vi "Dashboard Main.vi"() -> ()   [LabVIEW 2015]
uses:
  <vilib>/Utility/miscctls.llb/LVRowAndColumnTypeDef.ctl
  <vilib>/event_ctls.llb/eventvkey.ctl
  <vilib>/Rock Robotics/WPI/Dashboard/WPI_DashboardLogging Global.vi
  <vilib>/Rock Robotics/Network Tables/NT Read Numeric Array.vi
  <vilib>/Rock Robotics/Network Tables/NT Write Boolean.vi
  <vilib>/Utility/config.llb/Write Key (String).vi
  <vilib>/Utility/config.llb/Write Key (I32).vi
  <vilib>/Utility/config.llb/NI_LVConfig.lvlib
panel:
  in  "TCP":refnum<k5>
  in  "Rec Mode":enum32{"Stop", "Record", "Playback"}(radio)
  in  "Vision":u16(ring) items=["Camera Off", "USB Camera SW", "USB Camera HW", "IP Camera"]
  out "Camera IP":string
  out "Image Message":string="Timeout in Camera Communications"
  in  "Dashboard Tab":T1(tab)
  out "RPMs":dbl
  in  "Select Auto":string(combo)
  out "NT Connection":bool
  in  "Camera Settings":T2={"Frame Rate"=30, "Compression"=30, "Size"=1} {"Frame Rate" scale=1.0..30.0; "Size" items=["640x480", "320x240", "160x120"]}
  out "MotorChart R":cluster{"Numeric":dbl, "Numeric":dbl}(graph)
  out "MotorChart L":T3(graph)
  out "MotorSliders R":cluster{"MotorSlide1":dbl, "MotorSlide2":dbl} {"MotorSlide2" scale=-1.0..1.0 scale format="%#_2e"; "MotorSlide1" scale=-1.0..1.0 scale format="%#_2e"}
  out "MotorSliders L":T4 {"MotorSlide4 2" scale=0.0..14.0 scale format="%#_2e"; "MotorSlide2" scale=-1.0..1.0 scale format="%#_2e"; "MotorSlide1" scale=-1.0..1.0 scale format="%#_2e"}
  out "Gyro":dbl(knob) scale=0.0..360.0
  out "JS1 Z":dbl(slide) scale=-1.0..1.0 scale format="%#_2e"
  out "JS1 Graph":cluster{"X":dbl, "Y":dbl}[](graph)
  out "JS1 Buttons":T5
  out "JS2 Z":dbl(slide) scale=-1.0..1.0 scale format="%#_2e"
  out "JS2 Graph":cluster{"X":dbl, "Y":dbl}[](graph)
  out "JS2 Buttons":T5
  out "Mode":T6(ring)=enum."Auto Disabled"
  in  "DB Camera Config":bool
  out "fps":dbl format="%#.1g"
  out "Mbps":dbl format="%#.1g"
  out "Mbps LED":bool
  out "Particles (F)":dbl
  in  "Dispose Vision":bool
  out "Particles (M)":dbl
  in  "Load File":bool
  in  "Color Components":T7={"Hue"={8.0, 168.0}, "Sat"={21.0, 255.0}, "Val"={229.0, 255.0}} {"Val" scale=0.0..255.0; "Sat" scale=0.0..255.0; "Hue" scale=0.0..255.0 scale format="%#_3g"}
  in  "DB/String 9":string
  in  "DB/String 8":string
  in  "DB/String 7":string
  in  "DB/String 6":string
  in  "DB/String 5":string
  in  "DB/String 4":string
  in  "DB/String 3":string
  in  "DB/String 2":string
  in  "DB/String 1":string
  in  "DB/String 0":string
  in  "DB/Slider 0":dbl(slide) scale=0.0..5.0
  in  "DB/Slider 1":dbl(slide) scale=0.0..5.0
  in  "DB/Slider 2":dbl(slide) scale=0.0..5.0
  in  "DB/Slider 3":dbl(slide) scale=0.0..5.0
  out "DB/LED 3":bool
  out "DB/LED 2":bool
  out "DB/LED 1":bool
  out "DB/LED 0":bool
  in  "DB/Button 3":bool
  in  "DB/Button 2":bool
  in  "DB/Button 1":bool
  in  "DB/Button 0":bool caption="New Name"
  in  "Test Slider":dbl(slide) scale=0.0..100.0 scale format="%#_3g"
  in  "On/Off":bool caption="Solenoid"
  in  "Test Name":u16(ring) items=["Select the test to run..."]
  in  "Test Tree":string(tree)
  in  "Motor":cluster{"Value":dbl, "Enable":bool} {"Value" scale=-1.0..1.0 scale format="%#_3g"}
  out "Progress":T8 {"Test Progress" scale=0.0..100.0}
  in  "Rev/Fwd":cluster{"Forward":bool, "Reverse":bool}
  in  "Test Ring":u16(ring) items=["Monochrome", "Color"]
  out "Cmd Status":string
  in  "Execute Command":bool
  in  "Command Params":string[][](table)
  in  "Command Selection":i32(listbox)
  in  "CheckList":i32(listbox)
  out "Tree":string(tree)
  out "Camera Image":T9(plugin-control)
  out "Background":bool
  # "Left"
  # "Front"
  # "Right"
  # "Battery"
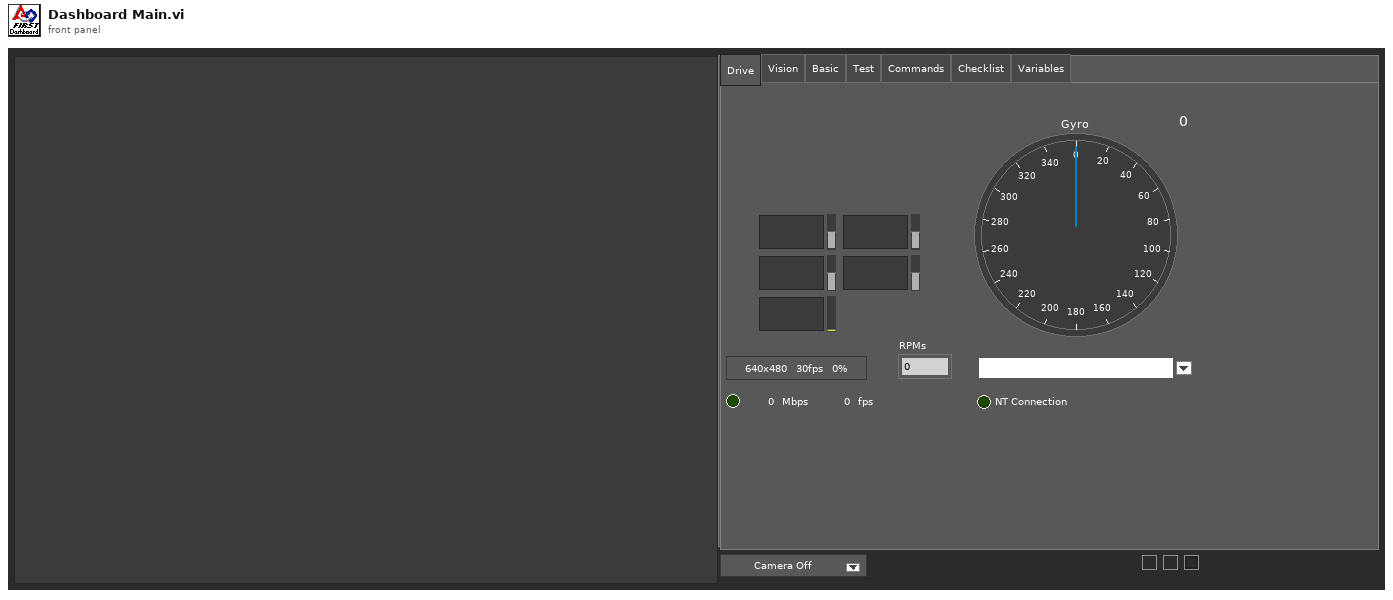
[diagram p1: front panel]
types:
  T1 = enum32{"Drive", "Vision", "Basic", "Test", "Commands", "Checklist", "Variables"}
  T2 = cluster{"Frame Rate":i32, "Compression":i32, "Size":u16}
  T3 = cluster{"Numeric":dbl, "Numeric":dbl, "Battery V":dbl}
  T4 = cluster{"MotorSlide1":dbl, "MotorSlide2":dbl, "MotorSlide4 2":dbl}
  T5 = cluster{bool, bool, bool, bool, bool, bool, bool, bool, bool, bool, bool, bool}
  T6 = enum8{"Tele-Op Disabled", "Tele-Op Enabled", "Auto Disabled", "Auto Enabled", "Test Disabled", "Test Enabled", "Disconnected", "No Code", "E-Stop"}
  T7 = cluster{"Hue":cluster{dbl, dbl}, "Sat":cluster{dbl, dbl}, "Val":cluster{dbl, dbl}}
  T8 = cluster{"Test Progress":u8, "Test Progress Text":string}
  T9 = typedef "IMAQ Image.ctl" = refnum<image>
  T10 = cluster{"IDs":cluster{"RPC field ID":u16, "Unique ID":u16}, "String":string}
  T11 = enum32{"Drive", "Basic", "Custom", "Test", "Checklist", "Variables"}
  T12 = typedef "Image Type" = u32
  T13 = cluster{"Camera Image":refnum<vi>, "Dashboard Tab":refnum<vi>, "Background":refnum<vi>, "Vision":refnum<vi>, "Rec Mode":refnum<vi>, "Test Slider":refnum<vi>, "On/Off ":refnum<vi>, "Test Ring":refnum<vi>, "Rev/Fwd":refnum<vi>, "Test Name":refnum<vi>, "Motor":refnum<vi>, "Progress":refnum<vi>, "CheckList":refnum<vi>, "Tree":refnum<vi>, "Test Tree":refnum<vi>, "Command Params":refnum<vi>, "Command Selection":refnum<vi>, "Execute Command":refnum<vi>, "Cmd Status":refnum<vi>}
  T14 = cluster{"Error Strings":string, "Disable Counts":cluster{u16, u16}, "Rail Faults":cluster{u16, u16, u16}, "Robot IP":string, "DB Mode":u8, "Event Info":cluster{"Name":string, "Type":u8, "Number":u16, "Replay":u8}, "Camera Addr":string}
  T15 = cluster{"Storage":cluster{"Disk Free":u64, "RAM Block":u32, "RAM free":u32}, "CPU Utilization":cluster{"CPU % ISR":sgl, "CPU % Time Crit":sgl, "CPU % Timed Str":sgl, "CPU % High":sgl, "CPU % Above":sgl, "CPU % Normal":sgl, "CPU % Low":sgl}, "CAN":cluster{"% Bus Utilization":sgl, "Bus Off Cnt":u32, "TX_FIFO Full Cnt":u32, "Receive Error Cnt":u8, "Transmit Error Cnt":u8}, "HID":cluster{"HID Outputs":u32, "Rumble Low":u16, "Rumble High":u16}[]}
  T16 = cluster{"Status bits":cluster{"Test Mode":bool, "Autonomous":bool, "Enabled":bool, "Code Start":bool, "Brownout":bool, "Reserved 2":bool, "Reserved 3":bool, "E-Stop":bool}, "Code Trace":cluster{"Disabled":bool, "TeleOp":bool, "Auto":bool, "Test":bool}, "Controller Type":enum16{"unknown", "cRIO", "roboRio"}, "Code?":enum16{"unknown", "noCode", "code"}, "Battery V":dbl}
  T17 = cluster{"Control Bits":cluster{"TestMode":bool, "Autonomous":bool, "Enabled":bool, "FMS Present":bool, bool, bool, bool, "E-Stop":bool}, "Team Station ":u8, "Countdown":sgl, "Joystick Values":cluster{"Axes":dbl[], "Buttons":bool[], "POVs":i16[]}[]}
  T18 = cluster{"Axes":dbl[], "Buttons":bool[], "POVs":i16[]}[]
  T19 = cluster{"Axes":dbl[], "Buttons":bool[], "POVs":i16[]}
  T20 = cluster{"Buttons[0]":bool, "Buttons[1]":bool, "Buttons[2]":bool, "Buttons[3]":bool, "Buttons[4]":bool, "Buttons[5]":bool, "Buttons[6]":bool, "Buttons[7]":bool, "Buttons[8]":bool, "Buttons[9]":bool, "Buttons[10]":bool, "Buttons[11]":bool}
  T21 = cluster{"Left":i32, "Top":i32, "Right":i32, "Bottom":i32}
  T22 = cluster{cluster{dbl, dbl}, cluster{dbl, dbl}, cluster{dbl, dbl}}
  T23 = typedef "NI_LVConfig.lvlib/Config Data RefNum.ctl" = refnum<k1>
  T24 = cluster{"Operation":enum16{"Update", "Clear"}, "Color Box":u32}[]
  T25 = typedef "eventvkey.ctl" = enum16{"ASCII", "Enter", "Return", "Shift", "Ctrl", "Alt", "Cmd", "Opt", "Caps", "NumLock", "Clear", "Break", "Up", "Down", "Left", "Right", "Insert", "Delete", "Home", "End", "PageUp", "PageDown", "Escape", "Help", "Pause", "ScrollLock", "F1", "F2", "F3", "F4", "F5", "F6", "F7", "F8", "F9", "F10", "F11", "F12", "F13", "F14", "F15", "F16", "F17", "F18", "F19", "F20", "F21", "F22", "F23", "F24", "Play", "VolumeUp", "VolumeDown", "Mute", "Two Byte Char"}
  T26 = cluster{"Image Size":bool, "Image Type":bool, "Pixel Value":bool, "ROI Information":bool, "Zoom Factor":bool}
  T27 = enum8{"Enabled", "Disabled", "Disabled and Grayed Out"}
  T28 = cluster{"Operation":enum16{"Update", "Clear"}, "Color Box":u32}
  T29 = typedef "LVRowAndColumnTypeDef.ctl" = cluster{"Row":i32, "Column":i32}
  T30 = cluster{"Shift":bool, "Ctrl":bool, "Alt":bool, "Cmd":bool, "Opt":bool}
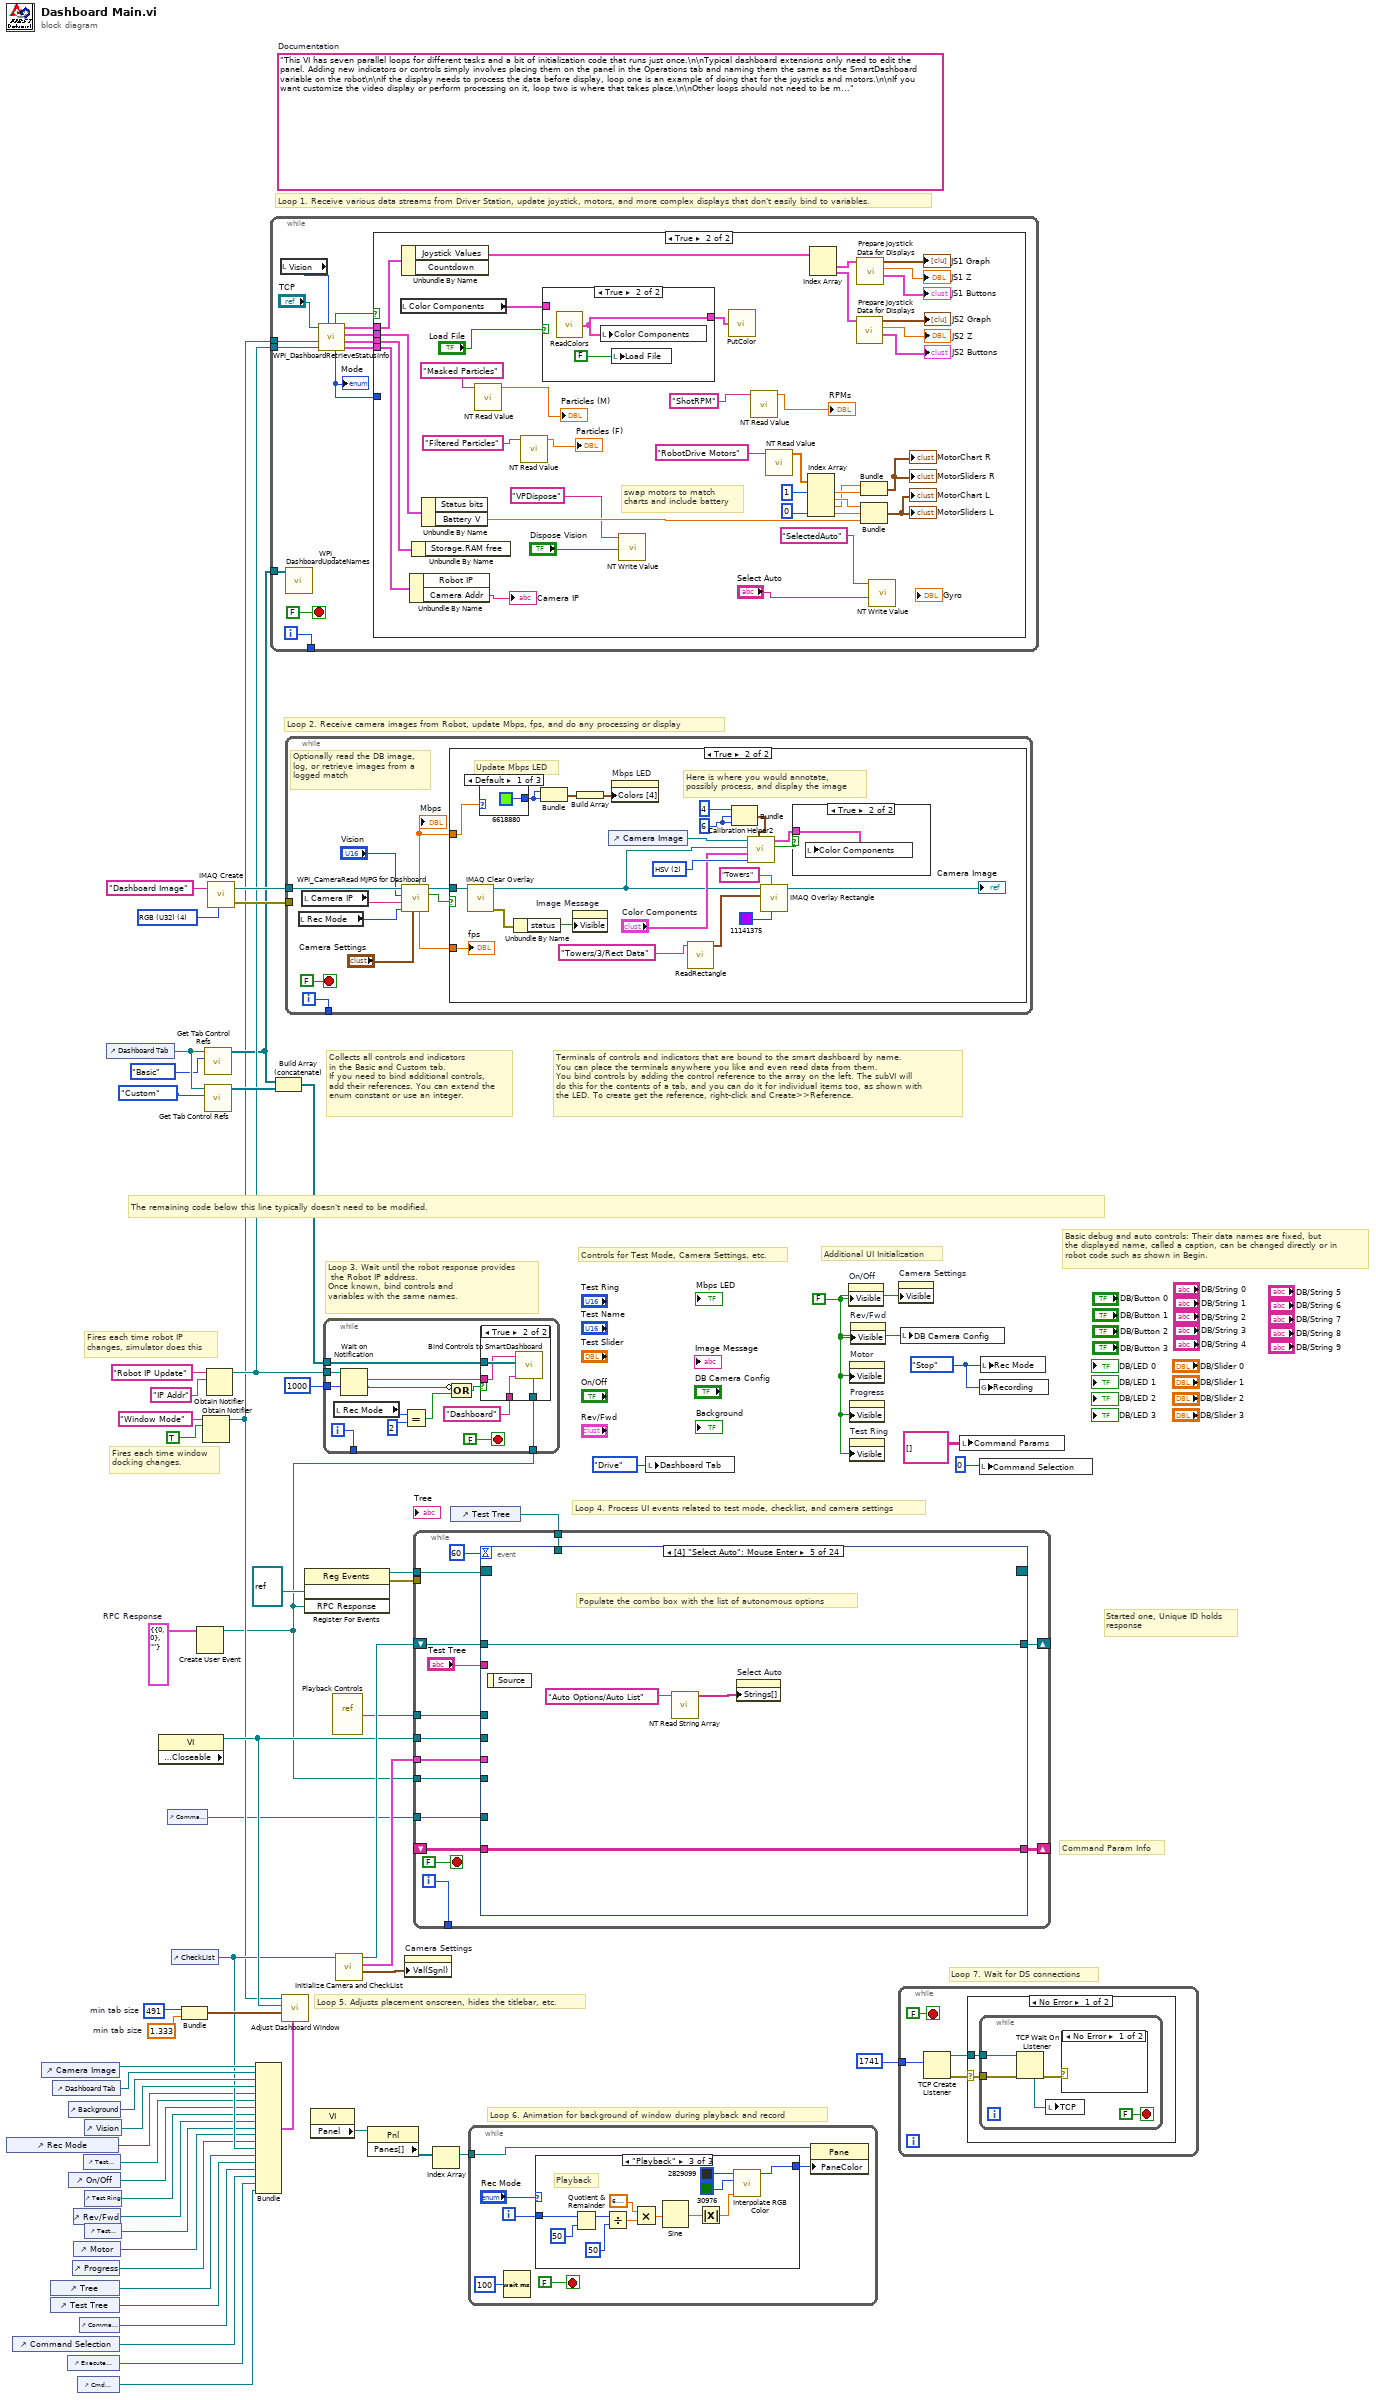
[diagram p0: block diagram]
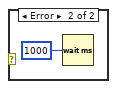
[diagram p2: hidden frame]
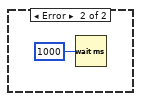
[diagram p3: hidden frame]
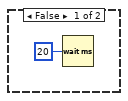
[diagram p4: hidden frame]
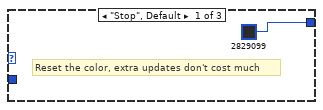
[diagram p6: hidden frame]
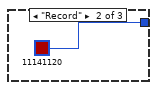
[diagram p7: hidden frame]
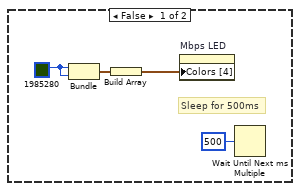
[diagram p9: hidden frame]
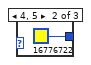
[diagram p11: hidden frame]
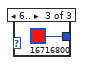
[diagram p12: hidden frame]
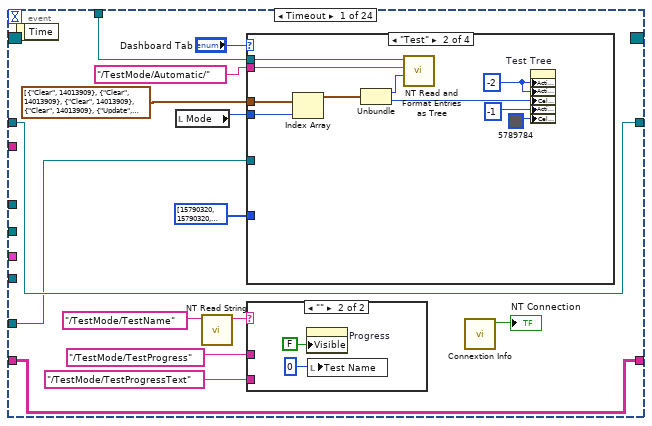
[diagram p13: hidden frame]
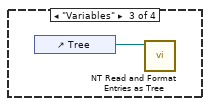
[diagram p15: hidden frame]
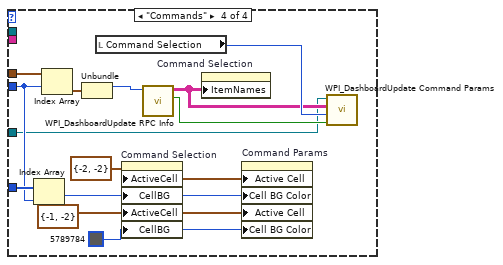
[diagram p16: hidden frame]
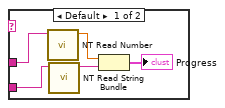
[diagram p17: hidden frame]
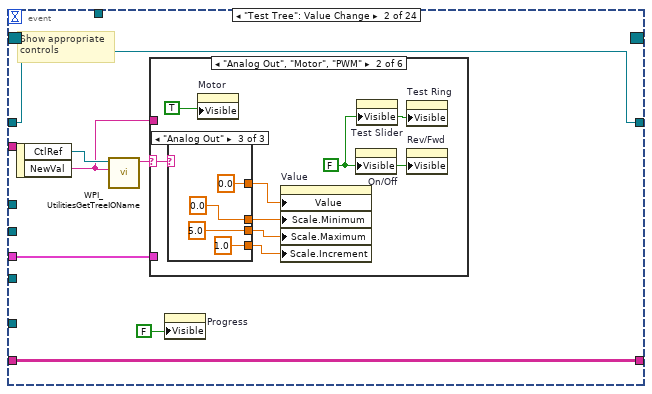
[diagram p18: hidden frame]
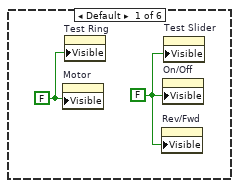
[diagram p19: hidden frame]
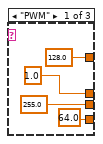
[diagram p20: hidden frame]
diagram:
  w8 = T10 {"IDs"={"RPC field ID"=0, "Unique ID"=0}, "String"=""}  # RPC Response
  w33 = 491  # min tab size
  w32 = 1.333  # min tab size
  w41 = enum32{"Stop", "Record", "Playback"}."Stop" ("Rec Mode")
  w15 = FALSE ("Visible")
  (unwired) "This VI has seven parallel loops for different tasks and a bit of initialization code that runs just once.\n\nTypical dashboard extensions only need to edit the panel. Adding new indicators or controls simply involves placing them on the panel in the Operations tab and naming them the same as the SmartDashboard variable on the robot\n\nIf the display needs to process the data before display, loop one is an example of doing that for the joysticks and motors.\n\nIf you want customize the video display or perform processing on it, loop two is where that takes place.\n\nOther loops should not need to be modified. They are pretty standard, and document the task they perform."  # Documentation
  w61 = T12 4 items=["Grayscale (U8)", "Grayscale (I16)", "Grayscale (SGL)", "Complex (CSG)", "RGB (U32)", "HSL (U32)", "RGB (U64)"] ("Image Type")
  # "Command Param Info"
  # "Started one, Unique ID holds\nresponse"
  # "Loop 7. Wait for DS connections"
  # "Basic debug and auto controls: Their data names are fixed, but\nthe displayed name, called a caption, can be changed directly or in\nrobot code such as shown in Begin."
  # "Controls for Test Mode, Camera Settings, etc."
  # "Additional UI Initialization"
  # "Loop 6. Animation for background of window during playback and record"
  # "Fires each time robot IP\nchanges, simulator does this"
  # "Fires each time window\ndocking changes."
  # "Collects all controls and indicators\nin the Basic and Custom tab.\nIf you need to bind additional controls,\nadd their references. You can extend the\nenum constant or use an integer."
  # "The remaining code below this line typically doesn't need to be modified."
  # "Loop 4. Process UI events related to test mode, checklist, and camera settings"
  # "Terminals of controls and indicators that are bound to the smart dashboard by name.\nYou can place the terminals anywhere you like and even read data from them.\nYou bind controls by adding the control reference to the array on the left. The subVI will\ndo this for the contents of a tab, and you can do it for individual items too, as shown with\nthe LED. To create get the reference, right-click and Create>>Reference."
  # "Loop 3. Wait until the robot response provides\n the Robot IP address.\nOnce known, bind controls and\nvariables with the same names."
  # "Loop 5. Adjusts placement onscreen, hides the titlebar, etc."
  # "Loop 1. Receive various data streams from Driver Station, update joystick, motors, and more complex displays that don't easily bind to variables."
  # "Loop 2. Receive camera images from Robot, update Mbps, fps, and do any processing or display"
  n1 = control-ref of="Rec Mode"() -> (w21:refnum<vi>)
  n2 = control-ref of="Command Selection"() -> (w7:refnum<vi>)
  n3 = control-ref of="Camera Image"() -> (w36:refnum<vi>)
  n4 = control-ref of="Tree"() -> (w25:refnum<vi>)
  n5 = control-ref of="Test Tree"() -> (w24:refnum<vi>)
  n6 = control-ref of="Dashboard Tab"() -> (w35:refnum<vi>)
  n7 = control-ref of="Execute Command"() -> (w9:refnum<vi>)
  n8 = control-ref of="Background"() -> (w30:refnum<vi>)
  n9 = control-ref of="On/Off"() -> (w19:refnum<vi>)
  n10 = control-ref of="Progress"() -> (w16:refnum<vi>)
  n11 = control-ref of="Rev/Fwd"() -> (w17:refnum<vi>)
  n12 = control-ref of="Motor"() -> (w22:refnum<vi>)
  n13 = control-ref of="Cmd Status"() -> (w3:refnum<vi>)
  n14 = control-ref of="Command Params"() -> (w10:refnum<vi>)
  n15 = control-ref of="Test Slider"() -> (w20:refnum<vi>)
  n16 = control-ref of="Vision"() -> (w34:refnum<vi>)
  n17 = control-ref of="Test Ring"() -> (w18:refnum<vi>)
  n18 = control-ref of="Test Name"() -> (w23:refnum<vi>)
  n19 = control-ref of="Dashboard Tab"() -> (w39:refnum<vi>)
  n20 = property class="VI" props=["Front Panel.Closeable"]() -> (reference out=w40:refnum<vi>)  [unwired: 2 in, 2 out]
  n21 = control-ref of="Command Params"() -> (w2:refnum<vi>)
  n22 = control-ref of="CheckList"() -> (w26:refnum<vi>)
  n23 = Bundle("min tab size"=w33, "min tab size"=w32) -> (w31:cluster{"min tab size":i32, "min tab size":dbl})  [unwired: 1 in]
  n24 = Create User Event(user event datatype=w8) -> (user event=w4:refnum<user-event>)  [unwired: 1 in, 1 out]
  n25 = Obtain Notifier(name (unnamed)="Window Mode", notification data type=TRUE) -> (notifier out=w12:refnum<notifier>)  [unwired: 2 in, 2 out]
  n26 = call <vilib>:"Get Tab Control Refs.vi"("Page Index"=T11."Basic" ("Dashboard Tab"), "TabControl in"=w39) -> ("ControlsOnPage"=w13:refnum<vi>[])  [unwired: 9 in]
  n27 = call <vilib>:"Get Tab Control Refs.vi"("Page Index"=T11."Custom" ("Dashboard Tab"), "TabControl in"=w39) -> ("ControlsOnPage"=w38:refnum<vi>[])  [unwired: 9 in]
  n28 = Obtain Notifier(name (unnamed)="Robot IP Update", notification data type="IP Addr" ("name (unnamed)")) -> (notifier out=w14:refnum<notifier>)  [unwired: 2 in, 2 out]
  n29 = call "IMAQ Create"("Image Name"="Dashboard Image", "Image Type"=w61) -> ("New Image"=w59:T9, "error out"=w58:errorcluster)  [unwired: 2 in, 1 out]
  n30 = Bundle("Camera Image"=w36, "Dashboard Tab"=w35, "Background"=w30, "Vision"=w34, "Rec Mode"=w21, "Test Slider"=w20, "On/Off"=w19, "Test Ring"=w18, "Rev/Fwd"=w17, "Test Name"=w23, "Motor"=w22, "Progress"=w16, "CheckList"=w26, "Tree"=w25, "Test Tree"=w24, "Command Params"=w10, "Command Selection"=w7, "Execute Command"=w9, "Cmd Status"=w3) -> (w27:T13)  [unwired: 1 in]
  n31 = while {
    tunnel: [w73] -> _
    tunnel: w14 -> [w67]
    tunnel: w13 -> [w66]
    tunnel: w12 -> [w62]
    i -> [w73]
    stop <- FALSE stop-if-true
    n32 = local read "Vision"() -> (w64:u16)
    n33 = call <vilib>:"WPI_DashboardUpdateNames.vi"("Controls on Tab"=w66) -> ()  [unwired: 11 in]
    n34 = call <vilib>:"WPI_DashboardRetrieveStatusInfo.vi"("Vision"=w64, "Binding Refnum"=w67, "Window Mode Notifier"=w62, "TCP Cnx"="TCP") -> ("Power and Errors"=w68:T14, "Robot Metrics"=w71:T15, "Status Info"=w72:T16, "Control Info"=w69:T17, "Robot Mode"=w65:T6, "Process?"=w70:bool)  [unwired: 2 in]
    "Mode" <- w65
    n35 = case shown="True" w70 {
      tunnel: w72 -> [_ w113]
      tunnel: w71 -> [_ w112]
      tunnel: w69 -> [_ w111]
      tunnel: w68 -> [_ w110]
      tunnel: w65 -> [_ _]
      frame False {
        n36 = Wait (ms)(milliseconds to wait=u32 20) -> ()  [unwired: 1 out]
      }
      frame True {
        # "swap motors to match\ncharts and include battery"
        n37 = local read "Color Components"() -> (w85:T7)
        n38 = Unbundle By Name(w111) -> ("Joystick Values"=w100:T18)  [unwired: 1 out]
        n39 = Unbundle By Name(w110) -> ("Camera Addr"=→"Camera IP":string)  [unwired: 1 out]
        n40 = Unbundle By Name(w112) -> ()  [unwired: 1 out]
        n41 = Unbundle By Name(w113) -> ("Battery V"=w101:dbl)  [unwired: 1 out]
        n42 = call-poly <vilib>:"NT Read Value.vi"("Name"="Masked Particles") -> ("Numeric"=→"Particles (M)":dbl)  [unwired: 9 in, 1 out]
        n43 = call-poly <vilib>:"NT Read Value.vi"("Name"="Filtered Particles") -> ("Numeric"=→"Particles (F)":dbl)  [unwired: 9 in, 1 out]
        n44 = case shown="True" "Load File" {
          tunnel: [w114 w115] -> w86
          tunnel: w85 -> [w114 _]
          frame False {
          }
          frame True {
            n45 = call "ReadColors.vi"() -> ("Color Components"=w115:T7)
            n46 = local write "Color Components"(w115) -> ()
            n47 = local write "Load File"(FALSE) -> ()
          }
        }
        n48 = call-poly <vilib>:"NT Write Value.vi"("Boolean"="Dispose Vision", "Name"="VPDispose") -> ()  [unwired: 9 in, 1 out]
        n49 = call "PutColor.vi"("Color Components"=w86) -> ()
        n50 = call-poly <vilib>:"NT Read Value.vi"("Name"="ShotRPM") -> ("Numeric"=→"RPMs":dbl)  [unwired: 9 in, 1 out]
        n51 = call-poly <vilib>:"NT Read Value.vi"("Name"="RobotDrive Motors") -> ("Numeric Array"=w89:dbl[])  [unwired: 9 in, 1 out]
        n52 = Index Array(array=w89, index #1=1, index #4=0) -> (element #1=w105:dbl, element #2=w106:dbl, element #3=w104:dbl, element #4=w109:dbl)  [unwired: 2 in]
        n53 = Index Array(array=w100) -> (element #1=w99:T19, element #2=w94:T19)  [unwired: 2 in]
        n54 = call "Prepare Joystick Data for Displays.vi"("Joystick Values"=w94) -> ("Buttons"=→"JS2 Buttons":T20, "Z Axis"=→"JS2 Z":dbl, "Cartesian Data"=→"JS2 Graph":cluster{"X axis":dbl, "X axis":dbl}[])  [unwired: 8 in]
        n55 = call "Prepare Joystick Data for Displays.vi"("Joystick Values"=w99) -> ("Buttons"=→"JS1 Buttons":T20, "Z Axis"=→"JS1 Z":dbl, "Cartesian Data"=→"JS1 Graph":cluster{"X axis":dbl, "X axis":dbl}[])  [unwired: 8 in]
        n56 = Bundle("Numeric"=w104, "Numeric"=w105) -> (→"MotorChart R" →"MotorSliders R":cluster{"Numeric":dbl, "Numeric":dbl})  [unwired: 1 in]
        n57 = Bundle("Numeric"=w106, "Numeric"=w109, "Battery V"=w101) -> (→"MotorChart L" →"MotorSliders L":T3)  [unwired: 1 in]
        n58 = call-poly <vilib>:"NT Write Value.vi"("String"="Select Auto", "Name"="SelectedAuto") -> ()  [unwired: 9 in, 1 out]
      }
    }
  }
  n59 = Build Array (concatenate)(w13, w38) -> (w37:refnum<vi>[])
  n60 = call "Adjust Dashboard Window.vi"("Sizing Refnums"=w27, "Size Constraints"=w31, "VI"=w40, "WIn Mode"=w12) -> ()  [unwired: 8 in]
  n61 = while {
    tunnel: w59 -> [w125]
    tunnel: w58 -> [_]
    tunnel: [w126] -> _
    i -> [w126]
    stop <- FALSE stop-if-true
    # "Optionally read the DB image,\nlog, or retrieve images from a\nlogged match"
    n62 = local read "Rec Mode"() -> (w120:enum32{"Stop", "Record", "Playback"})
    n63 = local read "Camera IP"() -> (w118:string)
    n64 = call <vilib>:"WPI_CameraRead MJPG for Dashboard.vi"("Camera Settings"="Camera Settings", "Rec Mode"=w120, "Camera IP"=w118, "Camera Mode"="Vision", "Refnum in"=w125) -> ("Active"=w123:bool, "Refnum out"=w124:T9, "FPS"=w122:dbl, "Bandwidth (Mbps)"=w117:dbl)  [unwired: 3 in]
    "Mbps" <- w117
    n65 = case shown="True" w123 {
      tunnel: w124 -> [_ w148]
      tunnel: w117 -> [_ w147]
      tunnel: w122 -> [_ w146]
      frame False {
        w128 = u32 1985280 ("Color Box")
        # "Sleep for 500ms"
        n66 = Bundle("Color Box"=w128, "Color Box"=w128) -> (w130:cluster{"Color Box":u32, "Color Box":u32})  [unwired: 1 out]
        n67 = Build Array(w130) -> (w129:cluster{"Color Box":u32, "Color Box":u32}[])
        n68 = property on="Mbps LED" class="Bool (strict)"("Colors [4]"=w129) -> ()  [unwired: 2 in, 2 out]
        n69 = Wait Until Next ms Multiple(millisecond multiple=u32 500) -> ()  [unwired: 1 out]
      }
      frame True {
        w141 = 6
        w144 = u16 2 items=["RGB", "HSL", "HSV", "HSI", "CIE L*a*b*", "CIE XYZ"] ("Color Mode")
        # "Here is where you would annotate,\npossibly process, and display the image"
        # "Update Mbps LED"
        n70 = call "IMAQ Clear Overlay"("Image"=w148) -> ("error out"=w152:errorcluster, "Image Out"=w137:T9)  [unwired: 2 in, 7 out]
        n71 = case shown="Default" w147 {
          tunnel: [u32 6618880 ("Color Box") u32 16776722 ("Color Box") u32 16716800 ("Color Box")] -> w149
          frame Default {
          }
          frame 4, 5 {
          }
          frame 6.. {
          }
        }
        n72 = Unbundle By Name(w152) -> ("status"=w153:bool)
        n73 = Bundle("Color Box"=w149, "Color Box"=w149) -> (w151:cluster{"Color Box":u32, "Color Box":u32})  [unwired: 1 out]
        n74 = property on="Image Message" class="Str"("Visible"=w153) -> ()  [unwired: 2 in, 2 out]
        n75 = Build Array(w151) -> (w150:cluster{"Color Box":u32, "Color Box":u32}[])
        n76 = control-ref of="Camera Image"() -> (w145:refnum<vi>)
        n77 = property on="Mbps LED" class="Bool (strict)"("Colors [4]"=w150) -> ()  [unwired: 2 in, 2 out]
        n78 = call "ReadRectangle.vi"("Name"="Towers/3/Rect Data") -> ("Rectangle"=w134:T21)  [unwired: 10 in]
        n79 = Bundle(4, w141, w141) -> (w140:cluster{i32, i32, i32})  [unwired: 1 in]
        n80 = call "Calibration Helper2.vi"("Std Devs"=w140, "Color Mode"=w144, "Color Components"="Color Components", "Image"=w137, "Image Ctl Refnum"=w145) -> ("Changed"=w139:bool, "output color"=w138:T22)  [unwired: 5 in]
        n81 = call "IMAQ Overlay Rectangle"("Color"=u32 11141375, "Group"="Towers", "Rectangle"=w134, "Image"=w137) -> ("Image Out"=→"Camera Image":T9)  [unwired: 6 in, 1 out]
        n82 = case shown="True" w139 {
          tunnel: w138 -> [_ w154]
          frame False {
          }
          frame True {
            n83 = local write "Color Components"(w154) -> ()
          }
        }
        "fps" <- w146
      }
    }
  }
  n84 = register-events(refnum<vi> refnum, w4) -> (reference out=w45:refnum<event-registration>, error out=w44:errorcluster)  [unwired: 2 in]
  n85 = property class="VI"() -> ("Panel"=w48:refnum<vi>)  [unwired: 2 in, 2 out]
  n86 = while {
    tunnel: w37 -> [w170]
    tunnel: w14 -> [w168]
    tunnel: [w166] -> _
    tunnel: u32 1000 ("milliseconds to wait") -> [w165]
    tunnel: w4 -> [w158]
    i -> [w166]
    stop <- FALSE stop-if-true
    n87 = local read "Rec Mode"() -> (w161:enum32{"Stop", "Record", "Playback"})
    n88 = Wait on Notification(notifier=w168, timeout in ms (-1)=w165) -> (notification=w167:string, timed out?=w163:bool)  [unwired: 2 in, 2 out]
    n89 = Equal?(x=w161, y=u16 2 ("Rec Mode")) -> (x = y?=w162:bool)
    n90 = Compound Arithmetic op=OR(invert w163, w162) -> (w164:bool)
    n91 = case shown="True" w164 {
      tunnel: w170 -> [_ w174]
      tunnel: w167 -> [_ w173]
      tunnel: "Dashboard" -> [_ w172]
      tunnel: w158 -> [_ w171]
      frame False {
      }
      frame True {
        n92 = call <vilib>:"Bind Controls to SmartDashboard.vi"("RPC ref"=w171, "Client Name"=w172, "Bound Control Refs"=w174, "Server IP Address"=w173) -> ()  [unwired: 8 in]
      }
    }
  }
  n93 = vi-ref "Playback Controls.vi"() -> (w46:refnum<vi>)
  n94 = call "Initialize Camera and CheckList.vi"("ListBox in"=w26) -> ("Cluster"=w52:cluster{"value":i32, "value":i32, "index":i32}, "Array"=w53:cluster{string[]}[], "File Refnum"=w51:T23)  [unwired: 8 in]
  n95 = property class="Pnl"(reference=w48) -> ("Panes[]"=w49:refnum<vi>[])  [unwired: 1 in, 2 out]
  n96 = property on="Camera Settings" class="Clust (strict)"("Val(Sgnl)"=w52) -> ()  [unwired: 2 in, 2 out]
  n97 = Index Array(array=w49) -> (element=w47:refnum<vi>)  [unwired: 1 in]
  n98 = control-ref of="Test Tree"() -> (w50:refnum<vi>)
  n99 = while {
    tunnel: w53 -> [w186]
    shift-right: [w185] -> _
    shift-left: w51 -> [w184]
    tunnel: [w183] -> _
    tunnel: w50 -> [w182]
    tunnel: w46 -> [w181]
    tunnel: w45 -> [w180]
    tunnel: w44 -> [_]
    tunnel: w40 -> [w179]
    tunnel: w4 -> [w178]
    tunnel: w2 -> [w177]
    shift-right: [w176] -> _
    shift-left: _ -> [w175]
    i -> [w183]
    stop <- FALSE stop-if-true
    n100 = event shown="[4] \"Select Auto\": Mouse Enter" {
      selector: w180 -> [_ _ _ _ _ _ _ _ _ _ _ _ _ _ _ _ _ _ _ _ _ _ _ _]
      dyn-events: [_ _ _ _ _ _ _ _ _ _ _ _ _ _ _ _ _ _ w495 _ _ _ _ _] -> _
      timeout: u32 60 ("milliseconds to wait") -> [_ _ _ _ _ _ _ _ _ _ _ _ _ _ _ _ _ _ _ _ _ _ _ _]
      tunnel: w182 -> [w199 _ _ _ _ _ _ _ _ _ _ _ _ _ _ _ _ _ _ _ _ _ _ _]
      tunnel: "Test Tree" -> [_ _ _ _ _ _ _ _ _ _ _ _ _ w458 w467 w470 w475 w484 _ _ _ _ _ _]
      tunnel: w186 -> [_ w237 _ _ _ _ _ _ _ _ _ w420 w451 _ _ _ _ _ _ _ _ _ _ _]
      tunnel: [w196 w236 w340 w346 w356 w360 w366 w378 w386 w392 w405 w419 w444 w457 w465 w469 w474 w483 w497 w513 w515 w523 w534 w539] -> w185
      tunnel: w184 -> [w196 w236 w340 w346 w356 w360 w366 w378 w386 w392 w405 w418 w444 w457 w465 w469 w474 w483 w497 w513 w515 w523 w534 w539]
      tunnel: w181 -> [_ _ _ _ _ _ _ _ _ _ _ _ _ _ _ _ _ _ w498 _ w518 _ _ _]
      tunnel: w179 -> [_ _ _ _ _ _ _ _ _ _ _ _ _ _ _ _ _ _ w493 _ _ _ _ _]
      tunnel: w178 -> [_ _ _ _ _ _ _ _ _ _ _ _ _ _ _ _ _ _ w489 _ _ _ _ _]
      tunnel: w177 -> [w191 _ _ _ _ _ w364 _ _ _ _ _ _ _ _ _ _ _ _ _ _ _ _ _]
      tunnel: [w190 w235 w339 w345 w355 w361 w362 w372 w383 w391 w404 w417 w443 w456 w464 w468 w473 w482 w488 w511 w514 w519 w527 w540] -> w176
      tunnel: w175 -> [w190 w235 w339 w345 w355 w361 w362 _ _ w391 w404 w417 w443 w456 w464 w468 w473 w482 w488 w511 w514 w519 w527 w540]
      event Timeout {
        n101 = event-data() -> ()  [unwired: 1 in, 1 out]
        n102 = local read "Mode"() -> (w193:T6)
        n103 = call <vilib>:"NT Read String.vi"("Name"="/TestMode/TestName") -> ("String"=w202:string)  [unwired: 9 in, 1 out]
        n104 = case shown="\"Test\"" "Dashboard Tab" {
          tunnel: w199 -> [_ w213 _ _]
          tunnel: "/TestMode/Automatic/" ("Name Pattern") -> [_ w212 _ _]
          tunnel: T24 [{"Operation"=enum."Clear", "Color Box"=14013909}, {"Operation"=enum."Clear", "Color Box"=14013909}, {"Operation"=enum."Clear", "Color Box"=14013909}, {"Operation"=enum."Clear", "Color Box"=14013909}, {"Operation"=enum."Update", "Color Box"=14013909}, {"Operation"=enum."Update", "Color Box"=16777215}, {"Operation"=enum."Clear", "Color Box"=14013909}, {"Operation"=enum."Clear", "Color Box"=14013909}, {"Operation"=enum."Clear", "Color Box"=14013909}] -> [_ w205 _ w222]
          tunnel: w193 -> [_ w204 _ w221]
          tunnel: u32[] [15790320, 15790320, 15790320, 15790320, 16777215, 16777215, 15790320, 15790320, 15790320] -> [_ _ _ w227]
          tunnel: w191 -> [_ _ _ w215]
          frame "Vision", Default {
          }
          frame "Test" {
            w211 = -2 ("Active Item:Row Number")
            n105 = Index Array(array=w205, index=w204) -> (element=w206:T28)
            n106 = Unbundle(w206) -> ("Operation"=w207:enum16{"Update", "Clear"}, "Color Box"=w208:u32)
            n107 = call <vilib>:"NT Read and Format Entries as Tree.vi"("Operation"=w207, "Name Pattern"=w212, "Tree Refnum"=w213) -> ()  [unwired: 7 in, 2 out]
            n108 = property on="Test Tree" class="Tree (strict)"("Active Item Row Number"=w211, "ActiveColNum"=w211, "CellBG"=w208, "Active Item Row Number"=-1 ("Active Item:Row Number"), "CellBG"=u32 5789784 ("Color Box")) -> ()  [unwired: 2 in, 2 out]
          }
          frame "Variables" {
            n109 = control-ref of="Tree"() -> (w214:refnum<vi>)
            n110 = call <vilib>:"NT Read and Format Entries as Tree.vi"("Tree Refnum"=w214) -> ()  [unwired: 9 in, 2 out]
          }
          frame "Commands" {
            w223 = u32 5789784 ("Color Box")
            w224 = T29 {"Row"=-1, "Column"=-2} ("Active Cell:Active Cell")
            w226 = T29 {"Row"=-2, "Column"=-2} ("Active Cell:Active Cell")
            n111 = Index Array(array=w227, index=w221) -> (element=w225:u32)
            n112 = Index Array(array=w222, index=w221) -> (element=w220:T28)
            n113 = Unbundle(w220) -> ("Operation"=w219:enum16{"Update", "Clear"})  [unwired: 1 out]
            n114 = local read "Command Selection"() -> (w218:i32)
            n115 = property on="Command Selection" class="MCListbox (strict)"("ActiveCell"=w226, "CellBG"=w225, "ActiveCell"=w224, "CellBG"=w223) -> ()  [unwired: 2 in, 2 out]
            n116 = call <vilib>:"WPI_DashboardUpdate RPC Info.vi"("Operation"=w219) -> ("update"=w217:bool, "commands"=w216:string[][])  [unwired: 9 in]
            n117 = property on="Command Selection" class="MCListbox (strict)"("ItemNames"=w216) -> ()  [unwired: 2 in, 2 out]
            n118 = property on="Command Params" class="Tbl (strict)"("Active Cell"=w226, "Cell BG Color"=w225, "Active Cell"=w224, "Cell BG Color"=w223) -> ()  [unwired: 2 in, 2 out]
            n119 = call <vilib>:"WPI_DashboardUpdate Command Params.vi"("Update"=w217, "NewVal"=w218, "Commands"=w216, "Param Tbl"=w215) -> ()  [unwired: 7 in, 1 out]
          }
        }
        n120 = case shown="\"\"" w202 {
          tunnel: "/TestMode/TestProgress" ("Name") -> [w229 _]
          tunnel: "/TestMode/TestProgressText" ("Name") -> [w228 _]
          frame Default {
            n121 = call <vilib>:"NT Read Number.vi"("Name"=w229) -> ("Numeric"=w230:dbl)  [unwired: 9 in, 1 out]
            n122 = call <vilib>:"NT Read String.vi"("Name"=w228) -> ("String"=w231:string)  [unwired: 9 in, 1 out]
            n123 = Bundle("Numeric"=w230, "String"=w231) -> (→"Progress":cluster{"Numeric":dbl, "String":string})  [unwired: 1 in]
          }
          frame "" {
            n124 = property on="Progress" class="Clust (strict)"("Visible"=FALSE) -> ()  [unwired: 2 in, 2 out]
            n125 = local write "Test Name"(u16 0) -> ()
          }
        }
        n126 = call <vilib>:"Connextion Info.vi"() -> ("Connected"=→"NT Connection":bool)  [unwired: 10 in, 1 out]
      }
      event "Test Tree": Value Change {
        # "Show appropriate\ncontrols"
        n127 = event-data() -> ("CtlRef"=w240:refnum<vi>, "NewVal"=w238:string)  [unwired: 1 in]
        n128 = call <vilib>:"WPI_UtilitiesGetTreeIOName.vi"("NewVal"=w238, "TreeControl in"=w240) -> ("I/O Name"=w241:string)  [unwired: 9 in]
        n129 = case shown="\"Analog Out\", \"Motor\", \"PWM\"" w241 {
          selector: w241 -> [_ w248 _ w270 w279 _]
          tunnel: w238 -> [_ _ w267 w269 _ w286]
          tunnel: w237 -> [_ _ _ _ _ w285]
          frame Default {
            w243 = FALSE ("Visible")
            w242 = FALSE ("Visible")
            n130 = property on="Motor" class="Clust (strict)"("Visible"=w242) -> ()  [unwired: 2 in, 2 out]
            n131 = property on="Test Ring" class="Ring (strict)"("Visible"=w242) -> ()  [unwired: 2 in, 2 out]
            n132 = property on="Rev/Fwd" class="Clust (strict)"("Visible"=w243) -> ()  [unwired: 2 in, 2 out]
            n133 = property on="On/Off" class="Bool (strict)"("Visible"=w243) -> ()  [unwired: 2 in, 2 out]
            n134 = property on="Test Slider" class="Slide (strict)"("Visible"=w243) -> ()  [unwired: 2 in, 2 out]
          }
          frame "Analog Out", "Motor", "PWM" {
            w249 = FALSE ("Visible")
            n135 = case shown="\"Analog Out\"" w248 {
              tunnel: [1.0 ("Value") -1.0 ("Value") 0.0 ("Value")] -> w247
              tunnel: [255.0 ("Value") 1.0 ("Value") 5.0 ("Value")] -> w246
              tunnel: [128.0 ("Value") 0.0 ("Value") 0.0 ("Value")] -> w245
              tunnel: [64.0 ("Value") 0.5 ("Value") 1.0 ("Value")] -> w244
              frame "PWM" {
              }
              frame "Motor", Default {
              }
              frame "Analog Out" {
              }
            }
            n136 = property on="Motor" class="Clust (strict)"("Visible"=TRUE) -> ()  [unwired: 2 in, 2 out]
            n137 = property on="Value" class="Slide (strict)"("Value"=w245, "Scale.Minimum"=w247, "Scale.Maximum"=w246, "Scale.Increment"=w244) -> ()  [unwired: 2 in, 2 out]
            n138 = property on="On/Off" class="Bool (strict)"("Visible"=w249) -> ()  [unwired: 2 in, 2 out]
            n139 = property on="Test Slider" class="Slide (strict)"("Visible"=w249) -> ()  [unwired: 2 in, 2 out]
            n140 = property on="Test Ring" class="Ring (strict)"("Visible"=w249) -> ()  [unwired: 2 in, 2 out]
            n141 = property on="Rev/Fwd" class="Clust (strict)"("Visible"=w249) -> ()  [unwired: 2 in, 2 out]
          }
          frame "Servo" {
            w265 = FALSE ("Visible")
            n142 = call <vilib>:"NT Read Number.vi"("Name"=w267) -> ("Numeric"=w266:dbl)  [unwired: 9 in, 1 out]
            n143 = property on="Test Slider" class="Slide (strict)"("Visible"=TRUE, "Scale.Maximum"=170.0 ("Scale.Range:Maximum")) -> ()  [unwired: 2 in, 2 out]
            n144 = local write "Test Slider"(w266) -> ()
            n145 = property on="Motor" class="Clust (strict)"("Visible"=w265) -> ()  [unwired: 2 in, 2 out]
            n146 = property on="Rev/Fwd" class="Clust (strict)"("Visible"=w265) -> ()  [unwired: 2 in, 2 out]
            n147 = property on="On/Off" class="Bool (strict)"("Visible"=w265) -> ()  [unwired: 2 in, 2 out]
            n148 = property on="Test Ring" class="Ring (strict)"("Visible"=w265) -> ()  [unwired: 2 in, 2 out]
          }
          frame "Relay", "Solenoid" {
            w268 = FALSE ("Visible")
            n149 = property on="Motor" class="Clust (strict)"("Visible"=w268) -> ()  [unwired: 2 in, 2 out]
            n150 = property on="Test Slider" class="Slide (strict)"("Visible"=w268) -> ()  [unwired: 2 in, 2 out]
            n151 = Search and Replace String(input string=w269, search string="/Value  **", replace string="/Direction") -> (result string=w275:string)  [unwired: 5 in, 3 out]
            n152 = property on="Test Ring" class="Ring (strict)"("Visible"=w268) -> ()  [unwired: 2 in, 2 out]
            n153 = call <vilib>:"NT Read String.vi"("Name"=w275) -> ("String"=w273:string)  [unwired: 9 in, 1 out]
            n154 = Equal?(x="Both directions", y=w273) -> (x = y?=w271:bool)
            n155 = Not(x=w271) -> (.not. x?=w272:bool)
            n156 = property on="Rev/Fwd" class="Clust (strict)"("Visible"=w271) -> ()  [unwired: 2 in, 2 out]
            n157 = property on="On/Off" class="Bool (strict)"("Visible"=w272, "Caption.Text"=w270) -> ()  [unwired: 2 in, 2 out]
          }
          frame "Compressor", "Digital Out" {
            w278 = FALSE ("Visible")
            # "Get direction and finish"
            n158 = property on="Motor" class="Clust (strict)"("Visible"=w278) -> ()  [unwired: 2 in, 2 out]
            n159 = property on="Test Slider" class="Slide (strict)"("Visible"=w278) -> ()  [unwired: 2 in, 2 out]
            n160 = property on="Test Ring" class="Ring (strict)"("Visible"=w278) -> ()  [unwired: 2 in, 2 out]
            n161 = property on="On/Off" class="Bool (strict)"("Visible"=TRUE, "Caption.Text"=w279) -> ()  [unwired: 2 in, 2 out]
            n162 = property on="Rev/Fwd" class="Clust (strict)"("Visible"=FALSE) -> ()  [unwired: 2 in, 2 out]
          }
          frame "Camera" {
            n163 = call <vilib>:"Get Last Path Segment.vi"("String in"=w286) -> ("String out"=w287:string)  [unwired: 10 in]
            n164 = property on="On/Off" class="Bool (strict)"("Visible"=FALSE) -> ()  [unwired: 2 in, 2 out]
            n165 = property on="Motor" class="Clust (strict)"("Visible"=FALSE) -> ()  [unwired: 2 in, 2 out]
            n166 = property on="Rev/Fwd" class="Clust (strict)"("Visible"=FALSE) -> ()  [unwired: 2 in, 2 out]
            n167 = case shown="\"White Balance  **\"" w287 {
              tunnel: w286 -> [w293 w302 w311 w320 w329 _ w335]
              tunnel: w285 -> [w291 w299 w308 w317 w326 _ _]
              frame "Size  **" {
                n168 = Index Array(array=w291) -> (element=w290:cluster{string[]})  [unwired: 1 in]
                n169 = call <vilib>:"NT Read String.vi"("Name"=w293) -> ("String"=w292:string)  [unwired: 9 in, 1 out]
                n170 = Unbundle(w290) -> (w288:string[])
                n171 = Match First String(2:w288, 3:w292) -> (0:w289:i32)  [unwired: 1 out]
                n172 = property on="Test Ring" class="Ring (strict)"("Value"=w289, "Strings []"=w288) -> ()  [unwired: 2 in, 2 out]
                n173 = property on="Test Ring" class="Ring (strict)"("Visible"=TRUE) -> ()  [unwired: 2 in, 2 out]
                n174 = property on="Test Slider" class="Slide (strict)"("Visible"=FALSE) -> ()  [unwired: 2 in, 2 out]
              }
              frame "White Balance  **" {
                n175 = Index Array(array=w299, index=1) -> (element=w300:cluster{string[]})
                n176 = call <vilib>:"NT Read String.vi"("Name"=w302) -> ("String"=w301:string)  [unwired: 9 in, 1 out]
                n177 = Unbundle(w300) -> (w297:string[])
                n178 = Match First String(2:w297, 3:w301) -> (0:w296:i32)  [unwired: 1 out]
                n179 = property on="Test Ring" class="Ring (strict)"("Value"=w296, "Strings []"=w297) -> ()  [unwired: 2 in, 2 out]
                n180 = property on="Test Ring" class="Ring (strict)"("Visible"=TRUE) -> ()  [unwired: 2 in, 2 out]
                n181 = property on="Test Slider" class="Slide (strict)"("Visible"=FALSE) -> ()  [unwired: 2 in, 2 out]
              }
              frame "Exposure  **" {
                n182 = Index Array(array=w308, index=2) -> (element=w309:cluster{string[]})
                n183 = call <vilib>:"NT Read String.vi"("Name"=w311) -> ("String"=w310:string)  [unwired: 9 in, 1 out]
                n184 = Unbundle(w309) -> (w305:string[])
                n185 = Match First String(2:w305, 3:w310) -> (0:w306:i32)  [unwired: 1 out]
                n186 = property on="Test Ring" class="Ring (strict)"("Value"=w306, "Strings []"=w305) -> ()  [unwired: 2 in, 2 out]
                n187 = property on="Test Ring" class="Ring (strict)"("Visible"=TRUE) -> ()  [unwired: 2 in, 2 out]
                n188 = property on="Test Slider" class="Slide (strict)"("Visible"=FALSE) -> ()  [unwired: 2 in, 2 out]
              }
              frame "Exposure Priority  **" {
                n189 = Index Array(array=w317, index=3) -> (element=w318:cluster{string[]})
                n190 = call <vilib>:"NT Read String.vi"("Name"=w320) -> ("String"=w319:string)  [unwired: 9 in, 1 out]
                n191 = Unbundle(w318) -> (w314:string[])
                n192 = Match First String(2:w314, 3:w319) -> (0:w315:i32)  [unwired: 1 out]
                n193 = property on="Test Ring" class="Ring (strict)"("Value"=w315, "Strings []"=w314) -> ()  [unwired: 2 in, 2 out]
                n194 = property on="Test Ring" class="Ring (strict)"("Visible"=TRUE) -> ()  [unwired: 2 in, 2 out]
                n195 = property on="Test Slider" class="Slide (strict)"("Visible"=FALSE) -> ()  [unwired: 2 in, 2 out]
              }
              frame "Color Enable  **" {
                n196 = Index Array(array=w326, index=4) -> (element=w327:cluster{string[]})
                n197 = call <vilib>:"NT Read String.vi"("Name"=w329) -> ("String"=w328:string)  [unwired: 9 in, 1 out]
                n198 = Unbundle(w327) -> (w323:string[])
                n199 = Match First String(2:w323, 3:w328) -> (0:w324:i32)  [unwired: 1 out]
                n200 = property on="Test Ring" class="Ring (strict)"("Value"=w324, "Strings []"=w323) -> ()  [unwired: 2 in, 2 out]
                n201 = property on="Test Ring" class="Ring (strict)"("Visible"=TRUE) -> ()  [unwired: 2 in, 2 out]
                n202 = property on="Test Slider" class="Slide (strict)"("Visible"=FALSE) -> ()  [unwired: 2 in, 2 out]
              }
              frame Default {
                n203 = property on="Test Ring" class="Ring (strict)"("Visible"=FALSE) -> ()  [unwired: 2 in, 2 out]
                n204 = property on="Test Slider" class="Slide (strict)"("Visible"=FALSE) -> ()  [unwired: 2 in, 2 out]
              }
              frame "Brightness  **", "Color Level  **", "Compression  **", "FPS  **", "Sharpness  **" {
                n205 = call <vilib>:"NT Read Number.vi"("Name"=w335) -> ("Numeric"=w334:dbl)  [unwired: 9 in, 1 out]
                n206 = local write "Test Slider"(w334) -> ()
                n207 = property on="Test Slider" class="Slide (strict)"("Visible"=TRUE, "Scale.Maximum"=100.0 ("Scale.Range:Maximum")) -> ()  [unwired: 2 in, 2 out]
                n208 = property on="Test Ring" class="Ring (strict)"("Visible"=FALSE) -> ()  [unwired: 2 in, 2 out]
              }
            }
          }
        }
        n209 = property on="Progress" class="Clust (strict)"("Visible"=FALSE) -> ()  [unwired: 2 in, 2 out]
      }
      event "Test Name": Mouse Enter {
        # "Populate the ring with the list of tests"
        n210 = event-data() -> ()  [unwired: 1 in, 1 out]
        n211 = call <vilib>:"NT Read String Array.vi"("Name"="/TestMode/TestList") -> ("String Array"=w344:string[])  [unwired: 9 in, 1 out]
        n212 = Build Array (concatenate)("Select the test to run...", w344) -> (w343:string[])
        n213 = property on="Test Name" class="Ring (strict)"("Strings []"=w343) -> ()  [unwired: 2 in, 2 out]
      }
      event "Test Name": Value Change {
        w347 = FALSE ("Visible")
        # "Tell the robot the test name to run"
        n214 = event-data() -> ("NewVal"=w351:u16)  [unwired: 1 in]
        n215 = property on="Test Name" class="Ring (strict)"() -> ("Strings []"=w352:string[])  [unwired: 2 in, 2 out]
        n216 = local write "Progress"(T8 {"Test Progress"=0, "Test Progress Text"=""} ("Progress")) -> ()
        n217 = Index Array(array=w352, index=w351) -> (element=w350:string)
        n218 = call <vilib>:"NT Write String.vi"("String"=w350, "Name"="/TestMode/TestName") -> ()  [unwired: 9 in, 1 out]
        n219 = property on="Progress" class="Clust (strict)"("Visible"=TRUE) -> ()  [unwired: 2 in, 2 out]
        n220 = property on="Motor" class="Clust (strict)"("Visible"=w347) -> ()  [unwired: 2 in, 2 out]
        n221 = property on="Test Slider" class="Slide (strict)"("Visible"=w347) -> ()  [unwired: 2 in, 2 out]
        n222 = property on="On/Off" class="Bool (strict)"("Visible"=w347) -> ()  [unwired: 2 in, 2 out]
        n223 = property on="Rev/Fwd" class="Clust (strict)"("Visible"=w347) -> ()  [unwired: 2 in, 2 out]
        n224 = property on="Test Ring" class="Ring (strict)"("Visible"=w347) -> ()  [unwired: 2 in, 2 out]
      }
      event "Select Auto": Mouse Enter {
        # "Populate the combo box with the list of autonomous options"
        n225 = event-data() -> ()  [unwired: 1 in, 1 out]
        n226 = call <vilib>:"NT Read String Array.vi"("Name"="Auto Options/Auto List") -> ("String Array"=w354:string[])  [unwired: 9 in, 1 out]
        n227 = property on="Select Auto" class="CmbBox"("Strings[]"=w354) -> ()  [unwired: 2 in, 2 out]
      }
      event "Select Auto": Value Change {
        # "User modified the Auto Selection. Write to NT variable so robot knows."
        n228 = event-data() -> ("NewVal"=w358:string)  [unwired: 1 in]
        n229 = call <vilib>:"NT Write String.vi"("String"=w358, "Name"="Auto Selector") -> ()  [unwired: 9 in, 1 out]
      }
      event "Command Selection": Value Change {
        # "Get the params and show in table"
        n230 = event-data() -> ("NewVal"=w365:i32)  [unwired: 1 in]
        n231 = property on="Command Selection" class="MCListbox (strict)"() -> ("ItemNames"=w363:string[][])  [unwired: 2 in, 2 out]
        n232 = call <vilib>:"WPI_DashboardUpdate Command Params.vi"("NewVal"=w365, "Commands"=w363, "Param Tbl"=w364) -> ()  [unwired: 8 in, 1 out]
      }
      event "Execute Command": Value Change {
        # "Started one, Unique ID holds\nresponse"
        n233 = event-data() -> ()  [unwired: 1 in, 1 out]
        n234 = property on="Command Selection" class="MCListbox (strict)"() -> ("ItemNames"=w377:string[][])  [unwired: 2 in, 2 out]
        n235 = Index Array(array=w377, index (row)="Command Selection", index (col)=0) -> (element=w375:string)
        n236 = call <vilib>:"Invoke Commands.vi"("Command Params"="Command Params", "Function Name"=w375) -> ("Params"=w371:u8, "Started"=w370:bool)  [unwired: 7 in, 1 out]
        n237 = Array Subset(array="Command Params", length (row)=w371) -> (w372:string[][])  [unwired: 3 in]
        n238 = Select(t="Executing" ("Cmd Status"), s=w370, f="" ("Cmd Status")) -> (s? t:f=→"Cmd Status":string)
      }
      event "Command Selection": Double Click {
        n239 = event-data() -> ("Row"=w387:i32)  [unwired: 1 in]
        n240 = property on="Command Selection" class="MCListbox (strict)"() -> ("ItemNames"=w390:string[][])  [unwired: 2 in, 2 out]
        n241 = local read "Command Params"() -> (w385:string[][])
        n242 = Index Array(array=w390, index (row)=w387, index (col)=0) -> (element=w388:string)
        n243 = call <vilib>:"Invoke Commands.vi"("Command Params"=w385, "Function Name"=w388) -> ("Params"=w384:u8, "Started"=w379:bool)  [unwired: 7 in, 1 out]
        n244 = Array Subset(array=w385, length (row)=w384) -> (w383:string[][])  [unwired: 3 in]
        n245 = Select(t="Executing" ("Cmd Status"), s=w379, f="" ("Cmd Status")) -> (s? t:f=w380:string)
        n246 = local write "Cmd Status"(w380) -> ()
      }
      event "CheckList": Double Click {
        # "Shift clears all"
        # "Update symbols on the listbox"
        n247 = event-data() -> ("PlatMods.Shift"=w393:bool, "Row"=w395:i32)  [unwired: 1 in]
        n248 = case shown="True" w393 {
          tunnel: w395 -> [w399 _]
          tunnel: 1 -> [w398 _]
          frame False {
            n249 = property on="CheckList" class="LstBox (strict)"() -> ("Item Symbols"=w397:i32[])  [unwired: 2 in, 2 out]
            n250 = Replace Array Subset(array=w397, new element=w398, index=w399) -> (w396:i32[])
            n251 = property on="CheckList" class="LstBox (strict)"("Item Symbols"=w396) -> ()  [unwired: 2 in, 2 out]
          }
          frame True {
            w400 = 0 ("Top Row")
            n252 = property on="CheckList" class="LstBox (strict)"() -> ("Number of Rows"=w402:u32)  [unwired: 2 in, 2 out]
            n253 = Initialize Array(0, w402) -> (w401:i32[])
            n254 = property on="CheckList" class="LstBox (strict)"("Top Row"=w400, "Value"=w400, "Item Symbols"=w401) -> ()  [unwired: 2 in, 2 out]
          }
        }
      }
      event "CheckList": Key Down {
        # "Update symbols on the listbox\nLeft and right keys check and uncheck"
        n255 = event-data() -> ("VKey"=w407:T25)  [unwired: 1 in]
        n256 = case shown="\"Left\", \"Right\"" w407 {
          selector: w407 -> [w412 _]
          tunnel: eventvkey."Left" ("VKey") -> [w410 _]
          frame "Left", "Right" {
            n257 = Equal?(x=w410, y=w412) -> (x = y?=w411:bool)
            n258 = Select(t=0, s=w411, f=1) -> (s? t:f=w413:i32)
            n259 = property on="CheckList" class="LstBox (strict)"() -> ("Item Symbols"=w416:i32[])  [unwired: 2 in, 2 out]
            n260 = Replace Array Subset(array=w416, new element=w413, index="CheckList") -> (w415:i32[])
            n261 = property on="CheckList" class="LstBox (strict)"("Item Symbols"=w415) -> ()  [unwired: 2 in, 2 out]
          }
          frame Default {
          }
        }
      }
      event "DB Camera Config": Value Change {
        # "Show or hide the cluster of controls, store in ini file"
        n262 = event-data() -> ("NewVal"=w421:bool)  [unwired: 1 in]
        n263 = case shown="False" w421 {
          tunnel: w420 -> [w430 _]
          tunnel: [w423 w441] -> w419
          tunnel: w418 -> [w422 w441]
          frame False {
            w437 = "Camera"
            w440 = FALSE ("Visible")
            n264 = local read "Camera Settings"() -> (w429:T2)
            n265 = Index Array(array=w430) -> (element=w433:cluster{string[]})  [unwired: 1 in]
            n266 = Unbundle(w429) -> ("Frame Rate"=w428:i32, "Compression"=w427:i32, "Size"=w431:u16)
            n267 = Unbundle(w433) -> (w432:string[])
            n268 = Index Array(array=w432, index=w431) -> (element=w426:string)
            n269 = call-poly <vilib>:"Write Key.vi"("section"=w437, "value"=w426, "key"="Size", "refnum"=w422) -> ("refnum out"=w439:T23)  [unwired: 2 in, 5 out]
            n270 = call-poly <vilib>:"Write Key.vi"("section"=w437, "value"=w428, "key"="FrameRate", "refnum"=w439) -> ("refnum out"=w438:T23)  [unwired: 1 in, 6 out]
            n271 = property on="Camera Settings" class="Clust (strict)"("Visible"=w440) -> ()  [unwired: 2 in, 2 out]
            n272 = local write "DB Camera Config"(w440) -> ()
            n273 = call-poly <vilib>:"Write Key.vi"("section"=w437, "value"=w427, "key"="Compression", "refnum"=w438) -> ("refnum out"=w424:T23)  [unwired: 1 in, 6 out]
            n274 = call <vilib>:"Close Config Data.vi"("refnum"=w424) -> ("file path"=w425:path)  [unwired: 2 in, 8 out]
            n275 = call <vilib>:"Open Config Data.vi"("configuration file path"=w425) -> ("refnum"=w423:T23)  [unwired: 8 in, 2 out]
          }
          frame True {
            n276 = property on="Camera Settings" class="Clust (strict)"("Visible"=TRUE) -> ()  [unwired: 2 in, 2 out]
          }
        }
      }
      event "Camera Settings": Value Change {
        # "Update summary string when any elements of DB camera change"
        n277 = event-data() -> ("NewVal"=w455:T2)  [unwired: 1 in]
        n278 = Index Array(array=w451) -> (element=w450:cluster{string[]})  [unwired: 1 in]
        n279 = Unbundle(w455) -> ("Frame Rate"=w446:i32, "Compression"=w445:i32, "Size"=w448:u16)
        n280 = Unbundle(w450) -> (w449:string[])
        n281 = Index Array(array=w449, index=w448) -> (element=w447:string)
        n282 = Format Into String(format string="%s   %dfps   %d%%", w447, w446, w445) -> (resulting string=w452:string)  [unwired: 2 in, 1 out]
        n283 = Build Array(w452) -> (w453:string[])
        n284 = property on="DB Camera Config" class="Bool (strict)"("Strings [4]"=w453) -> ()  [unwired: 2 in, 2 out]
      }
      event "Motor.Enable": Value Change {
        # "When the test mode otor enable helper is set, update that\ntree row item's value"
        n285 = event-data() -> ("NewVal"=w462:bool)  [unwired: 1 in]
        n286 = Unbundle("Motor") -> ("Value"=w461:dbl)  [unwired: 1 out]
        n287 = Select(t=w461, s=w462, f=0.0) -> (s? t:f=w459:dbl)
        n288 = call <vilib>:"NT Write Number.vi"("Numeric"=w459, "Name"=w458) -> ()  [unwired: 9 in, 1 out]
      }
      event "Test Slider": Value Change {
        # "When the test mode slider helper is set, update that\ntree row item's value"
        n289 = event-data() -> ("NewVal"=w466:dbl)  [unwired: 1 in]
        n290 = call <vilib>:"NT Write Number.vi"("Numeric"=w466, "Name"=w467) -> ()  [unwired: 9 in, 1 out]
      }
      event "On/Off": Value Change {
        # "When the test mode on/off helper value is set, update that\ntree row item's value"
        n291 = event-data() -> ("NewVal"=w472:bool)  [unwired: 1 in]
        n292 = Boolean To (0,1)(Boolean=w472) -> (0, 1=w471:i16)
        n293 = call <vilib>:"NT Write Number.vi"("Numeric"=w471, "Name"=w470) -> ()  [unwired: 9 in, 1 out]
      }
      event "Rev/Fwd": Value Change {
        # "When the test mode helper value for relays is set, update that\ntree row item's value"
        n294 = event-data() -> ("NewVal.Forward"=w481:bool, "NewVal.Reverse"=w480:bool)  [unwired: 1 in]
        n295 = Boolean To (0,1)(Boolean=w481) -> (0, 1=w477:i16)
        n296 = Boolean To (0,1)(Boolean=w480) -> (0, 1=w479:i16)
        n297 = Negate(x=w479) -> (-x=w478:i16)
        n298 = Add(x=w477, y=w478) -> (x+y=w476:i16)
        n299 = call <vilib>:"NT Write Number.vi"("Numeric"=w476, "Name"=w475) -> ()  [unwired: 9 in, 1 out]
      }
      event "Test Ring": Value Change {
        # "When a test mode helper value is selected from the ring,\nset the tree item's variable to the string value"
        n300 = event-data() -> ("NewVal"=w486:u16)  [unwired: 1 in]
        n301 = property on="Test Ring" class="Ring (strict)"() -> ("Strings []"=w487:string[])  [unwired: 2 in, 2 out]
        n302 = Index Array(array=w487, index=w486) -> (element=w485:string)
        n303 = call <vilib>:"NT Write String.vi"("String"=w485, "Name"=w484) -> ()  [unwired: 9 in, 1 out]
      }
      event "Rec Mode": Value Change {
        # "Update globals for recording mode and path to read log from.\nClear when logging and let NetworkTables set path for vision to\nuse."
        n304 = event-data() -> ("NewVal"=w499:enum32{"Stop", "Record", "Playback"})  [unwired: 1 in]
        n305 = global write "WPI_DashboardLogging Global.vi" "Logging Filename"(path "") -> ()
        n306 = global write "WPI_DashboardLogging Global.vi" "Recording"(w499) -> ()
        n307 = case shown="\"Playback\"" w499 {
          tunnel: w498 -> [_ w501 w510]
          tunnel: [_ _ w509] -> w495
          tunnel: [_ _ w508] -> _
          tunnel: w493 -> [_ _ w506]
          tunnel: cluster{i32, i32} {-250, 170} -> [_ _ w505]
          tunnel: [_ _ T26 {"Image Size"=TRUE, "Image Type"=TRUE, "Pixel Value"=TRUE, "ROI Information"=TRUE, "Zoom Factor"=FALSE} ("Image Information Shown:All Elements")] -> w491
          tunnel: [_ _ TRUE ("Zoom Factor")] -> w490
          tunnel: w489 -> [_ _ w502]
          frame Default {
          }
          frame "Stop", "Record" {
            # "Place Window too"
            n308 = invoke class="VI" method="FP.Close"(reference=w501) -> (reference out=w500:refnum<vi>)  [unwired: 2 in, 2 out]
            n309 = invoke class="VI" method="Abort VI"(reference=w500) -> ()  [unwired: 2 in, 3 out]
          }
          frame "Playback" {
            n310 = call "Open Playback Panel.vi"("Offset"=w505, "DB VI Ref"=w506, "Playback in"=w510) -> ("Playback out"=w507:refnum<vi>)  [unwired: 8 in]
            n311 = register-events(w507, w502) -> (reference out=w509:refnum<event-registration>, error out=w508:errorcluster)  [unwired: 2 in]
          }
        }
        n312 = property on="Camera Image" class="ImageControl"("Image Information Shown"=w491, "Image Information Visible"=w490) -> ()  [unwired: 2 in, 2 out]
        n313 = call <vilib>:"WPI_DashboardNT Log FieldName Cache.vi"("Operation"=enum16{"Lookup/Add", "Index", "Clear"}."Clear") -> ()  [unwired: 8 in, 3 out]
      }
      event Panel Close {
        w512 = enum32{"Stop", "Record", "Playback"}."Stop" ("Rec Mode")
        # "Playback window has been closed, abort"
        n314 = event-data() -> ()  [unwired: 1 in, 4 out]
        n315 = local write "Rec Mode"(w512) -> ()
        n316 = global write "WPI_DashboardLogging Global.vi" "Recording"(w512) -> ()
      }
      event Panel Close {
        # "Abort playback window and ourself"
        n317 = event-data() -> ()  [unwired: 1 in, 4 out]
        n318 = invoke class="VI" method="FP.Close"(reference=w518) -> (reference out=w517:refnum<vi>)  [unwired: 2 in, 2 out]
        n319 = invoke class="VI" method="Abort VI"(reference=w517) -> (error out=w516:errorcluster)  [unwired: 2 in, 2 out]
        n320 = invoke class="VI" method="Abort VI"(error in=w516) -> ()  [unwired: 2 in, 3 out]
      }
      event User Event {
        n321 = event-data() -> ("IDs"=w526:cluster{"RPC field ID":u16, "Unique ID":u16}, "String"=w525:string)  [unwired: 1 in]
        n322 = Bundle("IDs"=w526, "String"=w525) -> (w524:T10)  [unwired: 1 in]
        n323 = call <vilib>:"Retrieve RPC Response.vi"("RPC Response"=w524) -> ("Output"=w521:string[][])  [unwired: 10 in]
        n324 = Build Array (concatenate)(w519, w521) -> (w520:string[][])
        n325 = local write "Command Params"(w520) -> ()
        n326 = local write "Cmd Status"("" ("Cmd Status")) -> ()
      }
      event "Vision": Value Change {
        # "Enable/Disable Compression slider.\nHW USB is hard-coded into the camera"
        n327 = event-data() -> ("NewVal"=w533:u16)  [unwired: 1 in]
        n328 = Equal?(x=w533, y=u32 2 ("milliseconds to wait")) -> (x = y?=w531:bool)
        n329 = Select(t=T27."Disabled and Grayed Out" ("Disabled"), s=w531, f=T27."Enabled" ("Disabled")) -> (s? t:f=w528:T27)
        n330 = property on="Compression" class="Slide (strict)"("DisabledEnum"=w528) -> ()  [unwired: 2 in, 2 out]
      }
      event "Tree": Double Click {
        n331 = event-data() -> ("PlatMods"=w538:T30, "Tag"=w537:string)  [unwired: 1 in]
        n332 = Unbundle(w538) -> ("Shift"=w536:bool)  [unwired: 4 out]
        n333 = Not(x=w536) -> (.not. x?=w535:bool)
        n334 = call <vilib>:"NT Update Persistence.vi"("Persistence"=w535, "Name"=w537) -> ()  [unwired: 9 in, 1 out]
      }
    }
  }
  n335 = while {
    tunnel: w47 -> [w542]
    i -> [w545]
    stop <- FALSE stop-if-true
    n336 = Wait (ms)(milliseconds to wait=u32 100) -> ()  [unwired: 1 out]
    n337 = case shown="\"Playback\"" "Rec Mode" {
      tunnel: w545 -> [_ _ w560]
      tunnel: [u32 2829099 ("Base Color") u32 11141120 ("Target Color") w549] -> w541
      frame "Stop", Default {
        # "Reset the color, extra updates don't cost much"
      }
      frame "Record" {
      }
      frame "Playback" {
        # "Playback"
        n338 = Quotient & Remainder(x=w560, y=u32 50 ("milliseconds to wait")) -> (x-y*floor(x/y)=w556:u32)  [unwired: 1 out]
        n339 = Divide(x=w556, y=u32 50 ("milliseconds to wait")) -> (x/y=w553:dbl)
        n340 = Multiply(x=6.283185307179586, y=w553) -> (x*y=w558:dbl)
        n341 = Sine(x=w558) -> (sin(x)=w557:dbl)
        n342 = Absolute Value(x=w557) -> (abs(x)=w550:dbl)
        n343 = call "Interpolate RGB Color.vi"("Proportion"=w550, "Target Color"=u32 30976, "Base Color"=u32 2829099) -> ("Result Color"=w549:u32)  [unwired: 8 in]
      }
    }
    n344 = property class="Pane"(reference=w542, "PaneColor"=w541) -> ()  [unwired: 1 in, 2 out]
  }
  n345 = local write "Dashboard Tab"(T1."Drive" ("Dashboard Tab")) -> ()
  n346 = property on="On/Off" class="Bool (strict)"("Visible"=w15) -> ()  [unwired: 2 in, 2 out]
  n347 = property on="Motor" class="Clust (strict)"("Visible"=w15) -> ()  [unwired: 2 in, 2 out]
  n348 = property on="Progress" class="Clust (strict)"("Visible"=w15) -> ()  [unwired: 2 in, 2 out]
  n349 = property on="Test Ring" class="Ring (strict)"("Visible"=w15) -> ()  [unwired: 2 in, 2 out]
  n350 = property on="Rev/Fwd" class="Clust (strict)"("Visible"=w15) -> ()  [unwired: 2 in, 2 out]
  n351 = property on="Camera Settings" class="Clust (strict)"("Visible"=w15) -> ()  [unwired: 2 in, 2 out]
  n352 = while {
    tunnel: u16 1741 ("timeout ms (25000)") -> [w562]
    stop <- FALSE stop-if-true
    n353 = TCP Create Listener(10:w562) -> (0:w561:errorcluster, 3:w563:refnum<k5>)  [unwired: 4 in, 1 out]
    n354 = case shown="No Error" w561 {
      selector: w561 -> [w565 _]
      tunnel: w563 -> [w566 _]
      frame No Error {
        n355 = while {
          tunnel: w566 -> [w569]
          tunnel: w565 -> [w568]
          stop <- FALSE stop-if-true
          n356 = TCP Wait On Listener(8:w568, 11:w569) -> (0:w570:errorcluster, 4:w571:refnum<k5>)  [unwired: 2 in, 3 out]
          n357 = local write "TCP"(w571) -> ()
          n358 = case shown="No Error" w570 {
            frame No Error {
            }
            frame Error {
              n359 = Wait (ms)(milliseconds to wait=u32 1000) -> ()  [unwired: 1 out]
            }
          }
        }
      }
      frame Error {
        n360 = Wait (ms)(milliseconds to wait=u32 1000) -> ()  [unwired: 1 out]
      }
    }
  }
  n361 = local write "DB Camera Config"(w15) -> ()
  n362 = local write "Command Params"(string[][] [] ("Command Params")) -> ()
  n363 = global write "WPI_DashboardLogging Global.vi" "Recording"(w41) -> ()
  n364 = local write "Command Selection"(u16 0 ("milliseconds to wait")) -> ()
  n365 = local write "Rec Mode"(w41) -> ()
